vi "OrderGraphMonotonousIncreasing.vi"(1 "Power Graph":cluster{dbl[], dbl[]}) -> (0 "Cluster":cluster{dbl[], dbl[]})   [LabVIEW 2019]
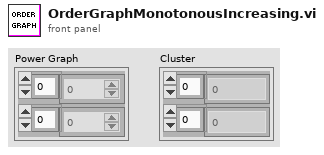
[diagram p1: front panel]
types:
  T1 = cluster{"Position Cached":dbl, "Power Cached":dbl}
  T2 = cluster{"Position Cached":dbl, "Power Cached":dbl}[]
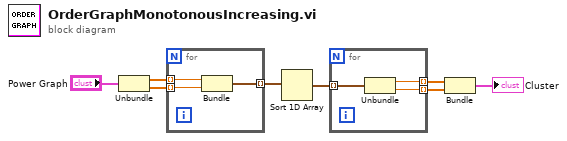
[diagram p0: block diagram]
diagram:
  n1 = Unbundle("Power Graph") -> (w7:dbl[], w6:dbl[])
  n2 = for {
    tunnel: w7 -> [w11] mode=indexing
    tunnel: w6 -> [w10] mode=indexing
    tunnel: [w9] -> w4 mode=indexing
    n3 = Bundle("Position Cached"=w11, "Power Cached"=w10) -> (w9:T1)  [unwired: 1 in]
  }
  n4 = Sort 1D Array(array=w4) -> (sorted array=w5:T2)
  n5 = for {
    tunnel: w5 -> [w14] mode=indexing
    tunnel: [w13] -> w1 mode=indexing
    tunnel: [w12] -> w8 mode=indexing
    n6 = Unbundle(w14) -> ("Position Cached"=w13:dbl, "Power Cached"=w12:dbl)
  }
  n7 = Bundle(w1, w8) -> (→"Cluster":cluster{dbl[], dbl[]})  [unwired: 1 in]
